vi "Constructor.vi"(7 "SQLite DB Path":path, 8 "error in (no error)":errorcluster {"code" format="Error %.0f"}, 11 "DBMap in":refnum<class "DBMap.lvclass">) -> (0 "error out":errorcluster {"code" format="Error %.0f"}, 3 "DBMap out":refnum<class "DBMap.lvclass">)   [LabVIEW 2020, in "DBMap.lvclass"]
uses:
  DBMap.lvclass
  DBMap.lvclass/DBMap.ctl
  <vilib>/drjdpowell/SQLite Library/SQL Connection/Connection.lvclass
  <vilib>/drjdpowell/SQLite Library/SQLite.lvlib
  <vilib>/drjdpowell/SQLite Library/SQL Connection/Open (string).vi
  <vilib>/drjdpowell/SQLite Library/SQL Connection/Execute SQL (No results).vi
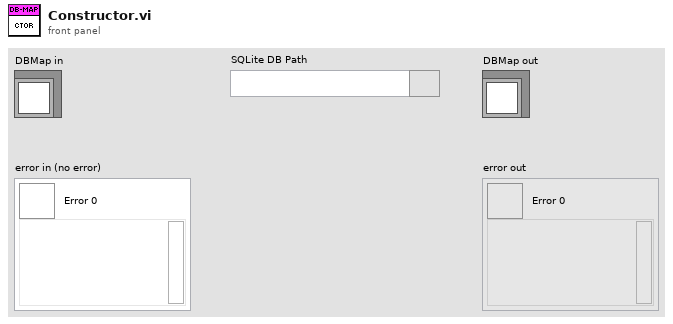
[diagram p1: front panel]
types:
  T1 = enum16{"New or existing", "Existing", "Read only"}
  T2 = typedef "Semaphore RefNum" = refnum<k1>
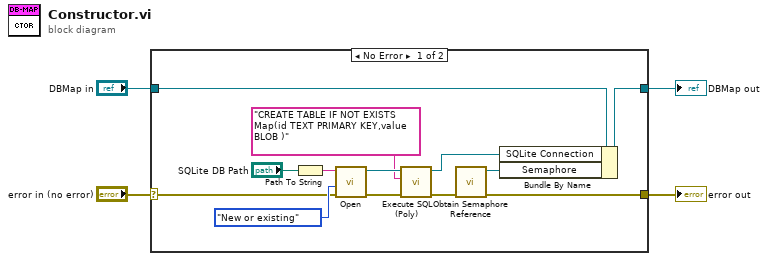
[diagram p0: block diagram]
diagram:
  n1 = case shown="No Error" "error in (no error)" {
    selector: "error in (no error)" -> [w11 w18]
    tunnel: "DBMap in" -> [w10 w19]
    tunnel: [w9 w19] -> w3
    tunnel: [w6 w18] -> w1
    frame No Error {
      n2 = Path To String(path="SQLite DB Path") -> (string=w15:string)
      n3 = call-poly <vilib>:"Open.vi"("error in (no error)"=w11, "File Option"=T1."New or existing", "db file"=w15) -> ("error out"=w16:errorcluster, "SQLite Connection"=w17:refnum<class "Connection.lvclass">)  [unwired: 7 in]
      n4 = call-poly <vilib>:"Execute SQL (Poly).vi"("error in (no error)"=w16, "SQL"="CREATE TABLE IF NOT EXISTS Map(id TEXT PRIMARY KEY,value BLOB )", "SQLite Connection in"=w17) -> ("error out"=w7:errorcluster, "SQLite Connection"=w8:refnum<class "Connection.lvclass">)  [unwired: 7 in]
      n5 = call <vilib>:"Obtain Semaphore Reference.vi"("error in (no error)"=w7) -> ("error out"=w6:errorcluster, "semaphore"=w5:T2)  [unwired: 4 in, 1 out]
      n6 = Bundle By Name(cluster=w10, "SQLite Connection"=w8, "Semaphore"=w5) -> (w9:refnum<class "DBMap.lvclass">)
    }
    frame Error {
    }
  }
  "error out" <- w1
  "DBMap out" <- w3
